vi "CreateDatabase.vi"(8 "错误输入（无错误）":errorcluster, 11 "测试类型":u16(ring) items=["温循", "高温老练", "常温拷机", "自定义测试", "单次测试", "自动测试"]) -> (0 "error out":errorcluster, 3 "数据库地址":string)   [LabVIEW 2014]
uses:
  <vilib>/addons/database/Connection.llb/DB Tools Open Connec (String).vi
  <vilib>/addons/database/Connection.llb/Conn Execute.vi
  <vilib>/addons/database/Recordset.llb/Rec Destroy - Connection.vi
  <vilib>/addons/database/NI_Database_API.lvlib
panel:
  out "连接的字符串 2":string
  in  "ADOX._Catalog":refnum<k7>
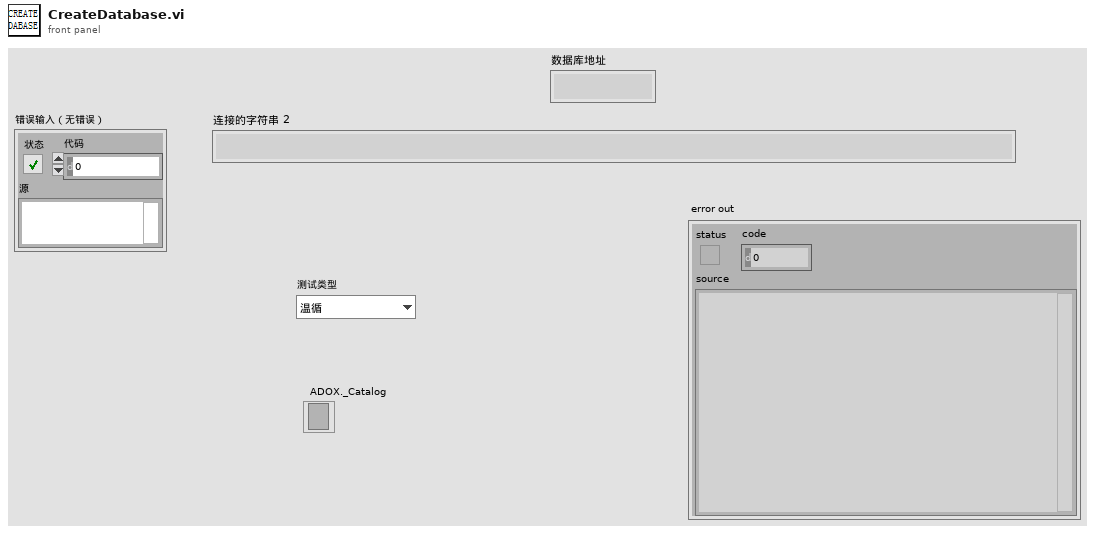
[diagram p1: front panel]
types:
  T1 = typedef "NI_Database_API.lvlib/Conn ObjectReference.ctl" = refnum<k1>
  T2 = typedef "NI_Database_API.lvlib/Rec ObjectReference.ctl" = refnum<k1>
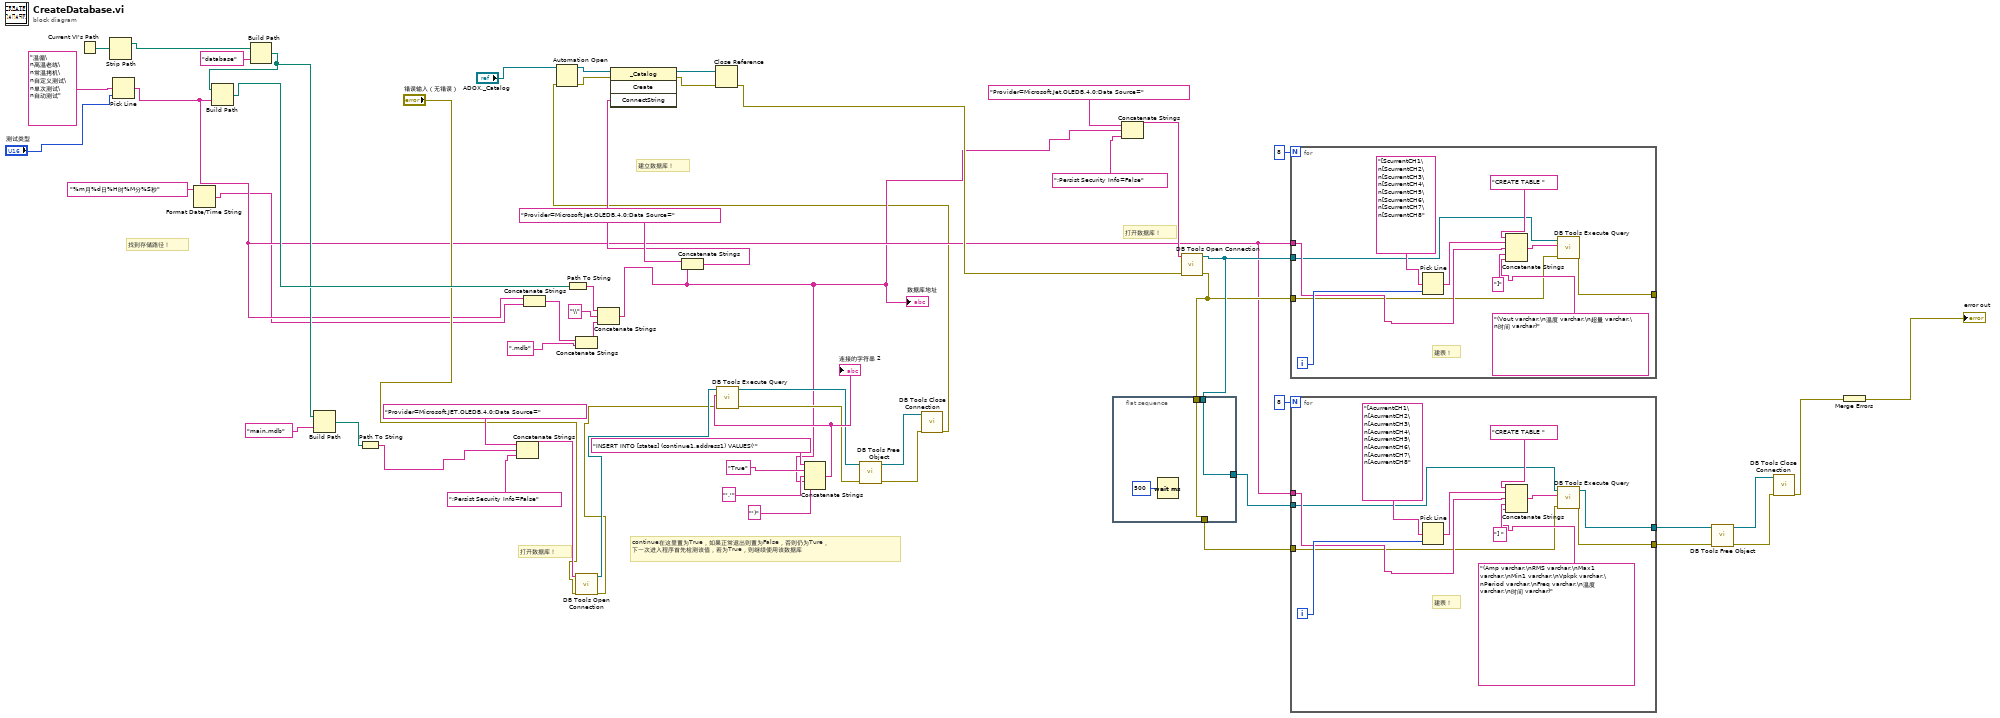
[diagram p0: block diagram]
diagram:
  # "打开数据库！"
  # "continue在这里置为True，如果正常退出则置为False，否则仍为Ture，\n下一次进入程序首先检测该值，若为True，则继续使用该数据库"
  # "打开数据库！"
  # "建立数据库！"
  # "找到存储路径！"
  n1 = Current VI's Path() -> (path=w47:path)
  n2 = Strip Path(path=w47) -> (stripped path=w46:path)  [unwired: 1 out]
  n3 = Pick Line(multi-line string="温循\n高温老练\n常温拷机\n自定义测试\n单次测试\n自动测试" ("多行字符串"), line index="测试类型") -> (output string=w7:string)  [unwired: 1 in]
  n4 = Format Date/Time String(time format string (%c)="%m月%d日%H时%M分%S秒" ("时间格式字符串(%c)")) -> (date/time string=w6:string)  [unwired: 2 in]
  n5 = Build Path(base path=w46, name or relative path="database" ("名称或相对路径")) -> (appended path=w18:path)
  n6 = Build Path(base path=w18, name or relative path=w7) -> (appended path=w39:path)
  n7 = Build Path(base path=w18, name or relative path="main.mdb" ("名称或相对路径")) -> (appended path=w16:path)
  n8 = Path To String(path=w16) -> (string=w15:string)
  n9 = Concatenate Strings("Provider=Microsoft.JET.OLEDB.4.0;Data Source=", w15, ";Persist Security Info=False") -> (w22:string)
  n10 = Concatenate Strings(w7, w6) -> (w3:string)
  n11 = Path To String(path=w39) -> (string=w43:string)
  n12 = Concatenate Strings(w3, ".mdb" ("字符串")) -> (w4:string)
  n13 = call-poly <vilib>:"DB Tools Open Connection.vi"("error in (no error)"="错误输入（无错误）", "connection information"=w22) -> ("error out"=w13:errorcluster, "connection reference"=w14:T1)  [unwired: 6 in]
  n14 = Concatenate Strings(w43, "\\" ("字符串"), w4) -> (w2:string)
  "数据库地址" <- w2
  n15 = Concatenate Strings("Provider=Microsoft.Jet.OLEDB.4.0;Data Source=", w2) -> (w52:string)
  n16 = Concatenate Strings("INSERT INTO [states] (continue1,address1) VALUES('", "True", "','", w2, "')") -> (w19:string)
  "连接的字符串 2" <- w19
  n17 = call-poly <vilib>:"DB Tools Execute Query.vi"("error in (no error)"=w13, "SQL query"=w19, "connection reference"=w14) -> ("error out"=w8:errorcluster, "recordset reference"=w9:T2)  [unwired: 5 in]
  n18 = call-poly <vilib>:"DB Tools Free Object.vi"("error in (no error)"=w8, "recordset reference"=w9) -> ("error out"=w10:errorcluster, "connection reference"=w11:T1)  [unwired: 8 in]
  n19 = call <vilib>:"DB Tools Close Connection.vi"("error in (no error)"=w10, "connection reference"=w11) -> ("error out"=w1:errorcluster)  [unwired: 5 in]
  n20 = Automation Open(error in (no error)=w1, Automation Refnum="ADOX._Catalog") -> (Automation Refnum=w57:refnum<k7>, error out=w56:errorcluster)  [unwired: 2 in]
  n21 = invoke class="_Catalog" method="Create"(reference=w57, error in=w56, "ConnectString"=w52) -> (reference out=w55:refnum<k7>, error out=w54:errorcluster)  [unwired: 1 in, 2 out]
  n22 = Close Reference(reference=w55, error in (no error)=w54) -> (error out=w48:errorcluster)
  n23 = flat-sequence {
    tunnel: w30 -> [w60]
    tunnel: [w60] -> w29
    tunnel: [w59] -> w27
    tunnel: w28 -> [w59]
    frame #0 {
      n24 = Wait (ms)(milliseconds to wait=u32 500 ("等待时间（毫秒）")) -> ()  [unwired: 1 out]
    }
  }
  n25 = Concatenate Strings("Provider=Microsoft.Jet.OLEDB.4.0;Data Source=", w2, ";Persist Security Info=False") -> (w49:string)
  n26 = call-poly <vilib>:"DB Tools Open Connection.vi"("error in (no error)"=w48, "connection information"=w49) -> ("error out"=w28:errorcluster, "connection reference"=w30:T1)  [unwired: 6 in]
  n27 = for {
    N: 8 -> [_]
    tunnel: [w67] -> _
    tunnel: w7 -> [w66]
    tunnel: w30 -> [w63]
    tunnel: w28 -> [w62]
    i -> [w69]
    # "建表！"
    n28 = Pick Line(multi-line string="[ScurrentCH1\n[ScurrentCH2\n[ScurrentCH3\n[ScurrentCH4\n[ScurrentCH5\n[ScurrentCH6\n[ScurrentCH7\n[ScurrentCH8" ("多行字符串"), line index=w69) -> (output string=w71:string)  [unwired: 1 in]
    n29 = Concatenate Strings("CREATE TABLE ", w71, w66, "]", "(Vout varchar,\n温度 varchar,\n超量 varchar,\n时间 varchar)") -> (w68:string)
    n30 = call-poly <vilib>:"DB Tools Execute Query.vi"("error in (no error)"=w62, "SQL query"=w68, "connection reference"=w63) -> ("error out"=w67:errorcluster)  [unwired: 5 in, 1 out]
  }
  n31 = for {
    N: 8 -> [_]
    tunnel: [w75] -> w33
    tunnel: [w79] -> w32
    tunnel: w7 -> [w78]
    tunnel: w29 -> [w74]
    tunnel: w27 -> [w73]
    i -> [w81]
    # "建表！"
    n32 = Pick Line(multi-line string="[AcurrentCH1\n[AcurrentCH2\n[AcurrentCH3\n[AcurrentCH4\n[AcurrentCH5\n[AcurrentCH6\n[AcurrentCH7\n[AcurrentCH8" ("多行字符串"), line index=w81) -> (output string=w83:string)  [unwired: 1 in]
    n33 = Concatenate Strings("CREATE TABLE ", w83, w78, "] ", "(Amp varchar,\nRMS varchar,\nMax1 varchar,\nMin1 varchar,\nVpkpk varchar,\nPeriod varchar,\nFreq varchar,\n温度 varchar,\n时间 varchar)") -> (w80:string)
    n34 = call-poly <vilib>:"DB Tools Execute Query.vi"("error in (no error)"=w73, "SQL query"=w80, "connection reference"=w74) -> ("error out"=w79:errorcluster, "recordset reference"=w75:T2)  [unwired: 5 in]
  }
  n35 = call-poly <vilib>:"DB Tools Free Object.vi"("error in (no error)"=w32, "recordset reference"=w33) -> ("error out"=w37:errorcluster, "connection reference"=w36:T1)  [unwired: 8 in]
  n36 = call <vilib>:"DB Tools Close Connection.vi"("error in (no error)"=w37, "connection reference"=w36) -> ("error out"=w35:errorcluster)  [unwired: 5 in]
  n37 = Merge Errors(w35) -> (→"error out":errorcluster)
